vi "ADCP_UI_Continuous_Transmitter.vi"(8 "error in (no error)":errorcluster, 11 "ADCU_GUI References":T1) -> ()   [LabVIEW 2017]
uses:
  Controls/ADCP_UI/ADCP_UI_Parameters.ctl
  Controls/ADCP_UI/ADCP_UI_Queues.ctl
  Controls/ADCP_UI/ADCP_UI_Continuous_Receiver_States.ctl
  Controls/ADCP_UI/ADCP_Queue_Receive_Log_Queue_Element.ctl
  Controls/Packet/Packet.ctl
  Controls/Packet/Packet_Direction.ctl
  Controls/Packet/Packet_Type.ctl
  Controls/Packet/Packet_Priority.ctl
  Controls/Data Packets/Data_Packet.ctl
  Controls/Data Packets/Parameter.ctl
  Controls/Data Packets/Parameter_Data_Type.ctl
  Controls/Data Packets/Data_Packet_Transmit_Mode.ctl
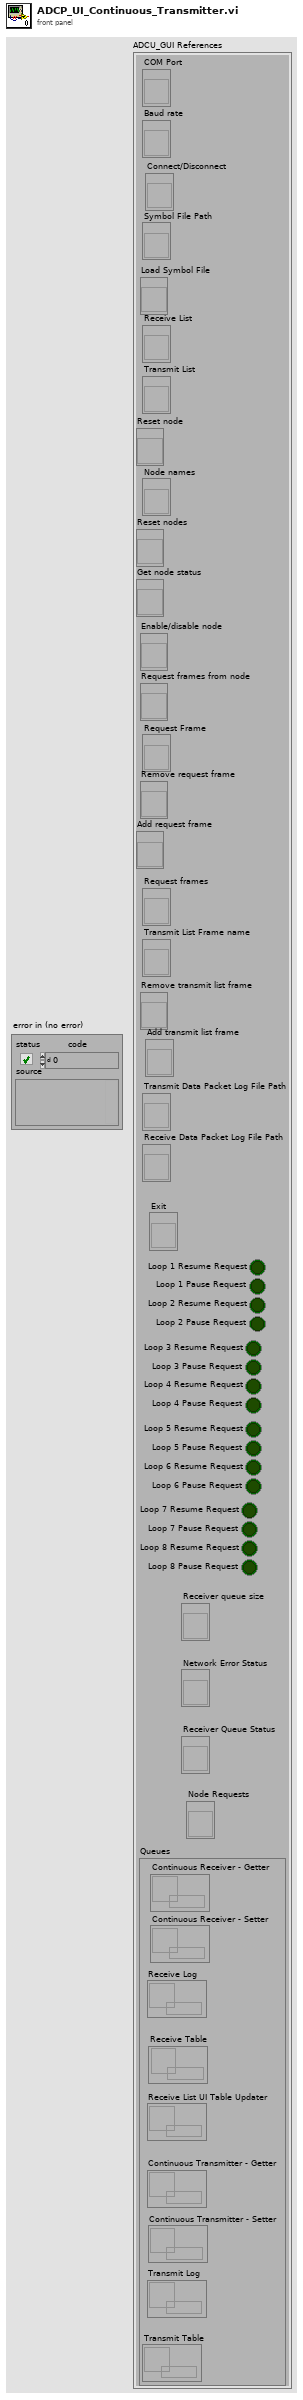
[diagram p1: front panel]
types:
  T1 = typedef "ADCP_UI_Parameters.ctl" = cluster{"COM Port":refnum<vi>, "Baud rate":refnum<vi>, "Symbol File Path":refnum<vi>, "Receive List":refnum<vi>, "Transmit List":refnum<vi>, "Node names":refnum<vi>, "Request Frame":refnum<vi>, "Request frames":refnum<vi>, "Transmit List Frame name":refnum<vi>, "Transmit Data Packet Log File Path":refnum<vi>, "Receive Data Packet Log File Path":refnum<vi>, "Loop 1 Resume Request":bool, "Loop 1 Pause Request":bool, "Loop 2 Resume Request":bool, "Loop 2 Pause Request":bool, "Loop 3 Resume Request":bool, "Loop 3 Pause Request":bool, "Loop 4 Resume Request":bool, "Loop 4 Pause Request":bool, "Loop 5 Resume Request":bool, "Loop 5 Pause Request":bool, "Loop 6 Resume Request":bool, "Loop 6 Pause Request":bool, "Loop 7 Resume Request":bool, "Loop 7 Pause Request":bool, "Loop 8 Resume Request":bool, "Loop 8 Pause Request":bool, "Exit":refnum<vi>, "Connect/Disconnect":refnum<vi>, "Load Symbol File":refnum<vi>, "Reset node":refnum<vi>, "Reset nodes":refnum<vi>, "Get node status":refnum<vi>, "Enable/disable node":refnum<vi>, "Request frames from node":refnum<vi>, "Remove request frame":refnum<vi>, "Add request frame":refnum<vi>, "Remove transmit list frame":refnum<vi>, "Add transmit list frame":refnum<vi>, "Receiver queue size":refnum<vi>, "Network Error Status":refnum<vi>, "Receiver Queue Status":refnum<vi>, "Node Requests":refnum<vi>, "Queues":T2}
  T2 = typedef "ADCP_UI_Queues.ctl" = cluster{"Continuous Receiver - Getter":refnum<queue>, "Continuous Receiver - Setter":refnum<queue>, "Receive Log":refnum<queue>, "Receive Table":refnum<queue>, "Receive List UI Table Updater":refnum<queue>, "Continuous Transmitter - Getter":refnum<queue>, "Continuous Transmitter - Setter":refnum<queue>, "Transmit Log":refnum<queue>, "Transmit Table":refnum<queue>}
  T3 = typedef "ADCP_UI_Continuous_Receiver_States.ctl" = enum16{"Disable", "Enable", "Exit"}
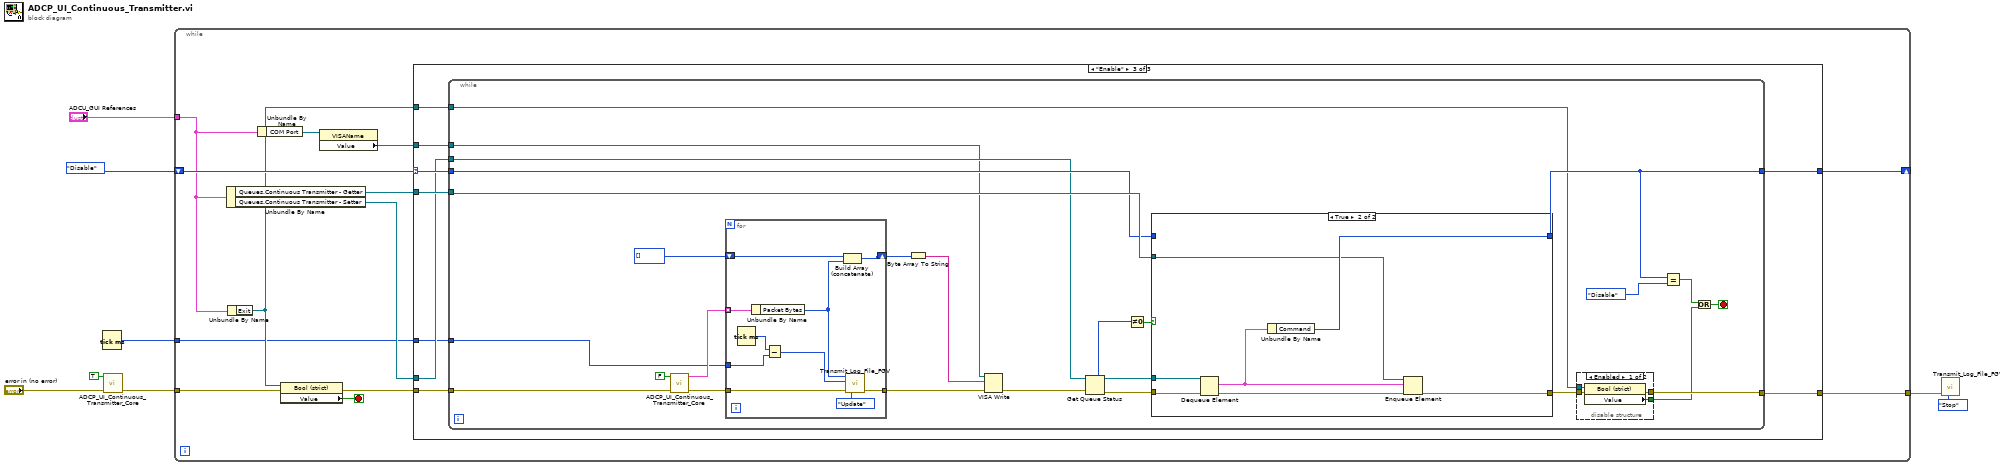
[diagram p0: block diagram]
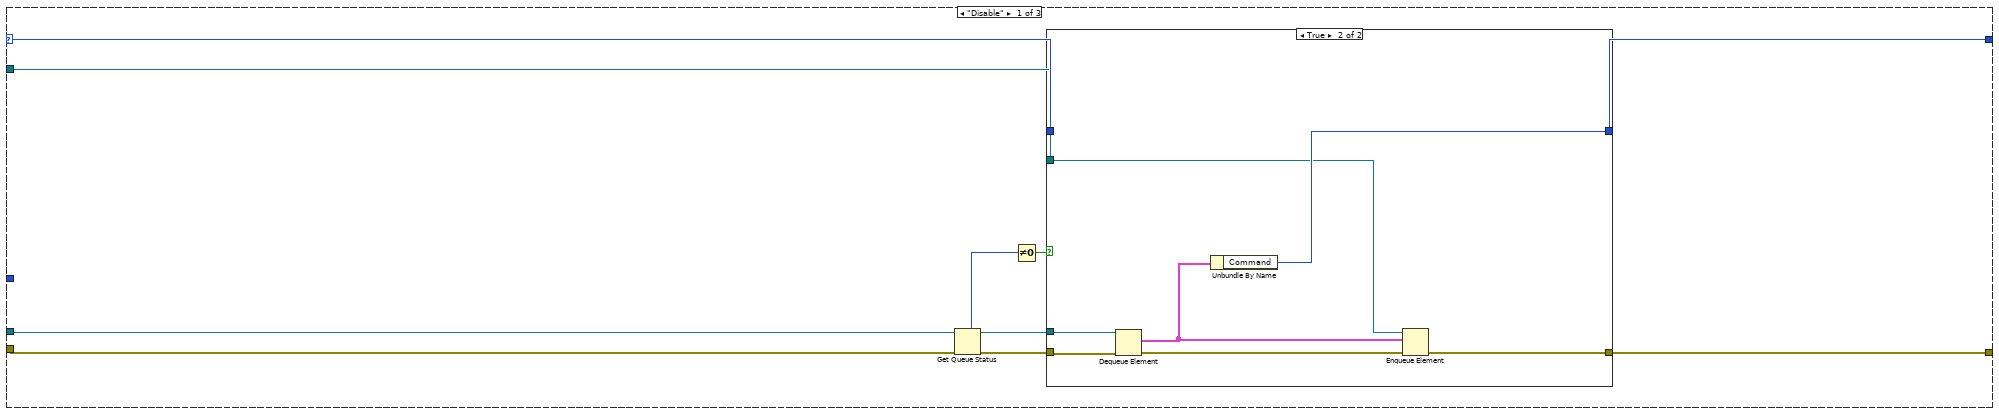
[diagram p2: hidden frame]
diagram:
  n1 = Tick Count (ms)() -> (millisecond timer value=w3:u32)
  n2 = call "ADCP_UI_Continuous_Transmitter_Core.vi"("error in (no error)"="error in (no error)", "Initialize ?"=TRUE) -> ("error out"=w5:errorcluster)  [unwired: 8 in, 1 out]
  n3 = while {
    tunnel: w5 -> [w21]
    shift-right: [w16] -> _
    shift-left: ADCP_UI_Continuous_Receiver_States."Disable" ("Enum") -> [w18]
    tunnel: "ADCU_GUI References" -> [w13]
    tunnel: [w15] -> w2
    tunnel: w3 -> [w9]
    stop <- w20 stop-if-true
    n4 = Unbundle By Name(w13) -> ("Queues.Continuous Transmitter - Getter"=w14:refnum<queue>, "Queues.Continuous Transmitter - Setter"=w17:refnum<queue>)
    n5 = Unbundle By Name(w13) -> ("Exit"=w10:refnum<vi>)
    n6 = Unbundle By Name(w13) -> ("COM Port"=w12:refnum<vi>)
    n7 = property class="Bool (strict)"(reference=w10, error in=w21) -> (error out=w19:errorcluster, "Value"=w20:bool)  [unwired: 1 out]
    n8 = property class="VISAName"(reference=w12) -> ("Value"=w11:refnum<visa-resource-name>)  [unwired: 1 in, 2 out]
    n9 = case shown="\"Enable\"" w18 {
      selector: w18 -> [w25 w42 w48]
      tunnel: w19 -> [w31 w41 w47]
      tunnel: w17 -> [w30 _ w46]
      tunnel: [w24 w42 w51] -> w16
      tunnel: [w23 w41 w50] -> w15
      tunnel: w14 -> [w22 _ w49]
      tunnel: w11 -> [_ _ w44]
      tunnel: w10 -> [_ _ w45]
      tunnel: w9 -> [_ _ w43]
      frame "Disable" {
        n10 = Get Queue Status(queue=w30, error in (no error)=w31) -> (queue out=w26:refnum<queue>, error out=w28:errorcluster, # elements in queue=w29:i32)  [unwired: 1 in, 5 out]
        n11 = Not Equal To 0?(x=w29) -> (x != 0?=w27:bool)
        n12 = case shown="True" w27 {
          tunnel: w28 -> [w32 w40]
          tunnel: w26 -> [_ w39]
          tunnel: [w33 w38] -> w24
          tunnel: w25 -> [w33 _]
          tunnel: [w32 w36] -> w23
          tunnel: w22 -> [_ w35]
          frame False {
          }
          frame True {
            n13 = Dequeue Element(queue=w39, error in (no error)=w40) -> (element=w34:cluster{"Command":T3, "Data":variant}, error out=w37:errorcluster)  [unwired: 1 in, 2 out]
            n14 = Unbundle By Name(w34) -> ("Command"=w38:T3)
            n15 = Enqueue Element(queue=w35, element=w34, error in (no error)=w37) -> (error out=w36:errorcluster)  [unwired: 1 in, 2 out]
          }
        }
      }
      frame "Exit" {
      }
      frame "Enable" {
        n16 = while {
          tunnel: [w71] -> w51
          tunnel: [w65] -> w50
          tunnel: w49 -> [w73]
          tunnel: w48 -> [w72]
          tunnel: w47 -> [w62]
          tunnel: w46 -> [w69]
          tunnel: w45 -> [w64]
          tunnel: w44 -> [w55]
          tunnel: w43 -> [w52]
          stop <- w68 stop-if-true
          n17 = call "ADCP_UI_Continuous_Transmitter_Core.vi"("error in (no error)"=w62, "Initialize ?"=FALSE) -> ("error out"=w60:errorcluster, "Packets"=w59:cluster{"Packet Bytes":u8[]}[])  [unwired: 8 in]
          n18 = for {
            tunnel: w60 -> [w82]
            tunnel: w59 -> [w87] mode=indexing
            shift-right: [w85] -> w54
            shift-left: u8[] [] -> [w86]
            tunnel: [w81] -> w57
            tunnel: w52 -> [w83]
            n19 = Tick Count (ms)() -> (millisecond timer value=w84:u32)
            n20 = Unbundle By Name(w87) -> ("Packet Bytes"=w80:u8[])
            n21 = Subtract(x=w84, y=w83) -> (x-y=w79:u32)
            n22 = Build Array (concatenate)(w86, w80) -> (w85:u8[])
            n23 = call "Transmit_Log_File_FGV.vi"("error in (no error)"=w82, "Command"=enum16{"Initialize", "Update", "Stop"}."Update", "Time (ms)"=w79, "Processed bytes"=w80) -> ("error out"=w81:errorcluster)  [unwired: 6 in, 1 out]
          }
          n24 = Byte Array To String(unsigned byte array=w54) -> (string=w53:string)
          n25 = VISA Write(VISA resource name=w55, write buffer=w53, error in (no error)=w57) -> (error out=w56:errorcluster)  [unwired: 2 out]
          n26 = Get Queue Status(queue=w69, error in (no error)=w56) -> (queue out=w74:refnum<queue>, error out=w76:errorcluster, # elements in queue=w77:i32)  [unwired: 1 in, 5 out]
          n27 = Not Equal To 0?(x=w77) -> (x != 0?=w75:bool)
          n28 = case shown="True" w75 {
            tunnel: w76 -> [w93 w101]
            tunnel: w74 -> [_ w100]
            tunnel: [w94 w99] -> w71
            tunnel: w72 -> [w94 _]
            tunnel: [w93 w97] -> w66
            tunnel: w73 -> [_ w96]
            frame False {
            }
            frame True {
              n29 = Dequeue Element(queue=w100, error in (no error)=w101) -> (element=w95:cluster{"Command":T3, "Data":variant}, error out=w98:errorcluster)  [unwired: 1 in, 2 out]
              n30 = Unbundle By Name(w95) -> ("Command"=w99:T3)
              n31 = Enqueue Element(queue=w96, element=w95, error in (no error)=w98) -> (error out=w97:errorcluster)  [unwired: 1 in, 2 out]
            }
          }
          n32 = disable-structure shown="Enabled" {
            disable-tunnel: w66 -> [w91 w92]
            disable-tunnel: [w90 w92] -> w65
            disable-tunnel: w64 -> [w89 _]
            disable-tunnel: [w88 _] -> w63
            frame Enabled {
              n33 = property class="Bool (strict)"(reference=w89, error in=w91) -> (error out=w90:errorcluster, "Value"=w88:bool)  [unwired: 1 out]
            }
            frame Disabled {
            }
          }
          n34 = Equal?(x=w71, y=ADCP_UI_Continuous_Receiver_States."Disable") -> (x = y?=w67:bool)
          n35 = Or(x=w67, y=w63) -> (x .or. y?=w68:bool)
        }
      }
    }
  }
  n36 = call "Transmit_Log_File_FGV.vi"("error in (no error)"=w2, "Command"=enum16{"Initialize", "Update", "Stop"}."Stop") -> ()  [unwired: 8 in, 2 out]
